vi "4155C Thermopower Heater ON Config SMUs.vi"(0 "VISA resource name in":refnum<visa-resource-name>, 1 "sweep method":u16(ring) items=["Continuous", "Pulsed"], 2 "Gate mode":u16(ring) items=["Auto", "Limited", "Fixed"], 3 "Gate Range":u8(slide)=6 max=11 scale=0.0..11.0, 5 "Pulse period":dbl=0.005 min=0.005 max=1.0 step=0.0001 format="%.4f", 7 "Pulse width":dbl=0.0005 min=0.0005 max=0.1 step=0.0001 format="%.4f", 8 "Drain Standby":bool, 9 "Base voltage":dbl format="%^.4e", 10 "Gate Standby":bool, 11 "error in (no error)":errorcluster, 12 "SMU4":cluster{"on/off":bool, "Voltage":dbl} {"Voltage" min=-100.0 max=100.0 format="%.2f"}, 13 "Source/drain mode":u16(ring) items=["Auto", "Limited", "Fixed"], 14 "Source/drain Range":u8(slide)=6 max=11 scale=0.0..11.0) -> (4 "VISA Resource Name out":refnum<visa-resource-name>, 15 "error out":errorcluster)   [LabVIEW 2016]
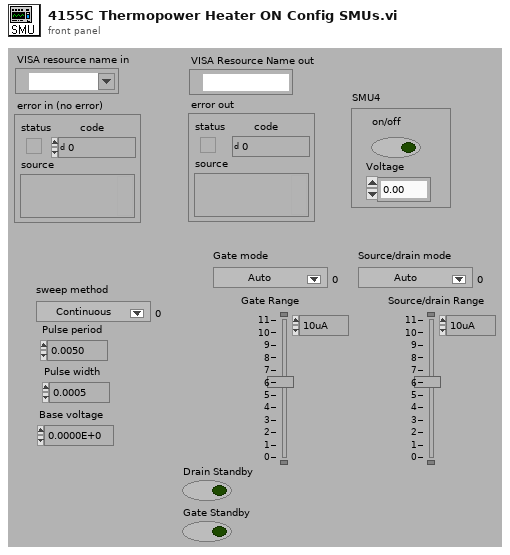
[diagram p1: front panel]
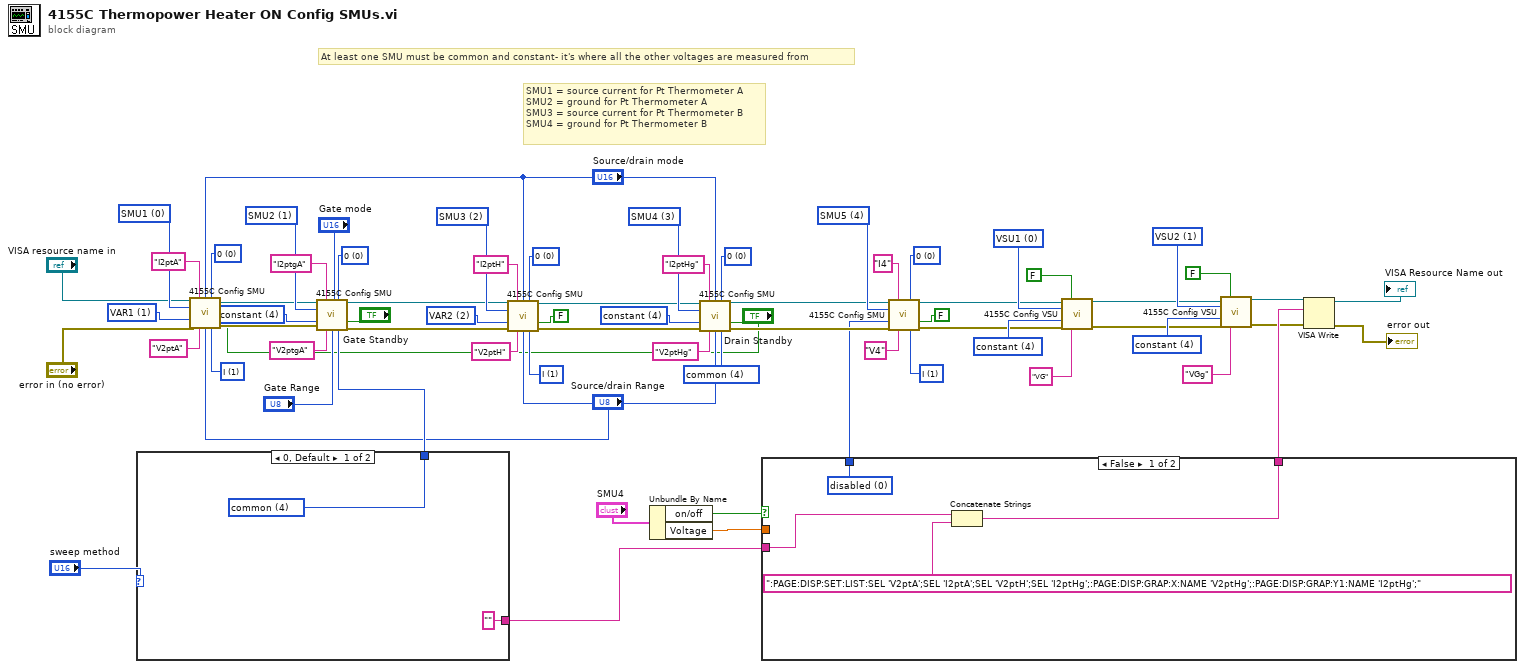
[diagram p0: block diagram]
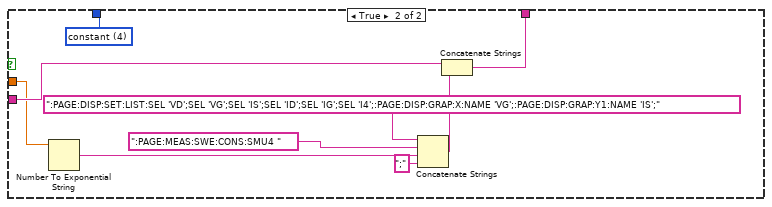
[diagram p2: hidden frame]
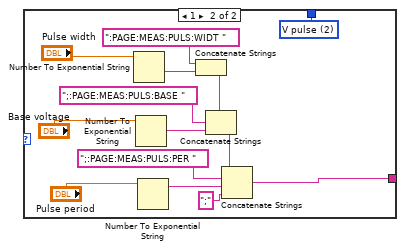
[diagram p3: hidden frame]
diagram:
  w7 = u32 4 items=["disabled  ", "VAR1  ", "VAR2  ", "VAR1'  ", "constant  "] ("function")
  w8 = u32 1 items=["VSU1  ", "VSU2  "] ("unit to configure")
  w13 = u32 4 items=["disabled  ", "VAR1  ", "VAR2  ", "VAR1'  ", "constant  "] ("function")
  w14 = u32 0 items=["VSU1  ", "VSU2  "] ("unit to configure")
  w29 = u32 0 items=["SMU1  ", "SMU2  ", "SMU3  ", "SMU4  ", "SMU5  ", "SMU6  "] ("unit to configure")
  w30 = u32 1 items=["disabled  ", "VAR1  ", "VAR2  ", "VAR1'  ", "constant  "] ("function")
  w32 = u32 0 items=["0  ", "10K Ohms  ", "100K Ohms  ", "1M Ohms  "] ("series resistance *")
  w33 = u32 1 items=["V  ", "I  ", "V pulse  ", "I pulse  ", "  common  "] ("mode")
  w49 = u32 1 items=["V  ", "I  ", "V pulse  ", "I pulse  ", "  common  "] ("mode")
  w50 = u32 0 items=["0  ", "10K Ohms  ", "100K Ohms  ", "1M Ohms  "] ("series resistance *")
  w52 = u32 4 items=["SMU1  ", "SMU2  ", "SMU3  ", "SMU4  ", "SMU5  ", "SMU6  "] ("unit to configure")
  w55 = u32 0 items=["0  ", "10K Ohms  ", "100K Ohms  ", "1M Ohms  "] ("series resistance *")
  w24 = u32 4 items=["disabled  ", "VAR1  ", "VAR2  ", "VAR1'  ", "constant  "] ("function")
  w57 = u32 1 items=["SMU1  ", "SMU2  ", "SMU3  ", "SMU4  ", "SMU5  ", "SMU6  "] ("unit to configure")
  w59 = u32 4 items=["V  ", "I  ", "V pulse  ", "I pulse  ", "  common  "] ("mode")
  w60 = u32 0 items=["0  ", "10K Ohms  ", "100K Ohms  ", "1M Ohms  "] ("series resistance *")
  w62 = u32 4 items=["disabled  ", "VAR1  ", "VAR2  ", "VAR1'  ", "constant  "] ("function")
  w63 = u32 3 items=["SMU1  ", "SMU2  ", "SMU3  ", "SMU4  ", "SMU5  ", "SMU6  "] ("unit to configure")
  w66 = u32 1 items=["V  ", "I  ", "V pulse  ", "I pulse  ", "  common  "] ("mode")
  w67 = u32 0 items=["0  ", "10K Ohms  ", "100K Ohms  ", "1M Ohms  "] ("series resistance *")
  w69 = u32 2 items=["disabled  ", "VAR1  ", "VAR2  ", "VAR1'  ", "constant  "] ("function")
  w70 = u32 2 items=["SMU1  ", "SMU2  ", "SMU3  ", "SMU4  ", "SMU5  ", "SMU6  "] ("unit to configure")
  # "SMU1 = source current for Pt Thermometer A\nSMU2 = ground for Pt Thermometer A\nSMU3 = source current for Pt Thermometer B\nSMU4 = ground for Pt Thermometer B"
  # "At least one SMU must be common and constant- it's where all the other voltages are measured from"
  n1 = case shown="0, Default" "sweep method" {
    tunnel: [w72 w86] -> w41
    tunnel: ["" w74] -> w21
    frame 0, Default {
      w72 = u32 4 items=["V  ", "I  ", "V pulse  ", "I pulse  ", "  common  "] ("mode")
    }
    frame 1 {
      w86 = u32 2 items=["V  ", "I  ", "V pulse  ", "I pulse  ", "  common  "] ("mode")
      n2 = Number To Exponential String(number="Pulse width") -> (E-format string=w82:string)  [unwired: 3 out]
      n3 = Number To Exponential String(number="Base voltage") -> (E-format string=w78:string)  [unwired: 3 out]
      n4 = Number To Exponential String(number="Pulse period") -> (E-format string=w75:string)  [unwired: 3 out]
      n5 = Concatenate Strings(":PAGE:MEAS:PULS:WIDT " ("Substring"), w82) -> (w80:string)
      n6 = Concatenate Strings(w80, ";:PAGE:MEAS:PULS:BASE " ("Substring"), w78) -> (w76:string)
      n7 = Concatenate Strings(w76, ";:PAGE:MEAS:PULS:PER " ("Substring"), w75, ";" ("Substring")) -> (w74:string)
    }
  }
  n8 = call "4155C Config SMU.vi"("VISA session"="VISA resource name in", "I name (max 6 chars)"="I2ptA", "Range mode"="Source/drain mode", "series resistance *"=w32, "unit to configure"=w29, "function"=w30, "standby"="Drain Standby", "error in (no error)"="error in (no error)", "V name (max 6 chars)"="V2ptA", "Range"="Source/drain Range", "mode"=w33) -> ("dup VISA resource name"=w27:refnum<visa-resource-name>, "error out"=w28:errorcluster)  [unwired: 3 out]
  n9 = call "4155C Config SMU.vi"("VISA session"=w27, "I name (max 6 chars)"="I2ptgA", "Range mode"="Gate mode", "series resistance *"=w55, "unit to configure"=w57, "function"=w24, "standby"="Gate Standby", "error in (no error)"=w28, "V name (max 6 chars)"="V2ptgA", "Range"="Gate Range", "mode"=w41) -> ("dup VISA resource name"=w38:refnum<visa-resource-name>, "error out"=w37:errorcluster)  [unwired: 3 out]
  n10 = call "4155C Config SMU.vi"("VISA session"=w38, "I name (max 6 chars)"="I2ptH", "Range mode"="Source/drain mode", "series resistance *"=w67, "unit to configure"=w70, "function"=w69, "standby"=FALSE, "error in (no error)"=w37, "V name (max 6 chars)"="V2ptH", "Range"="Source/drain Range", "mode"=w66) -> ("dup VISA resource name"=w46:refnum<visa-resource-name>, "error out"=w45:errorcluster)  [unwired: 3 out]
  n11 = Unbundle By Name("SMU4") -> ("on/off"=w19:bool, "Voltage"=w20:dbl)
  n12 = call "4155C Config SMU.vi"("VISA session"=w46, "I name (max 6 chars)"="I2ptHg", "Range mode"="Source/drain mode", "series resistance *"=w60, "unit to configure"=w63, "function"=w62, "standby"="Drain Standby", "error in (no error)"=w45, "V name (max 6 chars)"="V2ptHg", "Range"="Source/drain Range", "mode"=w59) -> ("dup VISA resource name"=w35:refnum<visa-resource-name>, "error out"=w36:errorcluster)  [unwired: 3 out]
  n13 = case shown="False" w19 {
    tunnel: w21 -> [w89 w99]
    tunnel: [w88 w98] -> w17
    tunnel: w20 -> [_ w96]
    tunnel: [w87 w97] -> w16
    frame False {
      w87 = u32 0 items=["disabled  ", "VAR1  ", "VAR2  ", "VAR1'  ", "constant  "] ("function")
      n14 = Concatenate Strings(w89, ":PAGE:DISP:SET:LIST:SEL 'V2ptA';SEL 'I2ptA';SEL 'V2ptH';SEL 'I2ptHg';:PAGE:DISP:GRAP:X:NAME 'V2ptHg';:PAGE:DISP:GRAP:Y1:NAME 'I2ptHg';" ("write buffer (\"\")")) -> (w88:string)
    }
    frame True {
      w97 = u32 4 items=["disabled  ", "VAR1  ", "VAR2  ", "VAR1'  ", "constant  "] ("function")
      n15 = Number To Exponential String(number=w96) -> (E-format string=w94:string)  [unwired: 3 out]
      n16 = Concatenate Strings(":PAGE:DISP:SET:LIST:SEL 'VD';SEL 'VG';SEL 'IS';SEL 'ID';SEL 'IG';SEL 'I4';:PAGE:DISP:GRAP:X:NAME 'VG';:PAGE:DISP:GRAP:Y1:NAME 'IS';" ("write buffer (\"\")"), ":PAGE:MEAS:SWE:CONS:SMU4 " ("write buffer (\"\")"), w94, ";" ("Substring")) -> (w92:string)
      n17 = Concatenate Strings(w99, w92) -> (w98:string)
    }
  }
  n18 = call "4155C Config SMU.vi"("VISA session"=w35, "I name (max 6 chars)"="I4", "series resistance *"=w50, "unit to configure"=w52, "function"=w16, "standby"=FALSE, "error in (no error)"=w36, "V name (max 6 chars)"="V4", "mode"=w49) -> ("dup VISA resource name"=w10:refnum<visa-resource-name>, "error out"=w9:errorcluster)  [unwired: 2 in, 3 out]
  n19 = call "4155C Config VSU.vi"("VISA session"=w10, "standby"=FALSE, "unit to configure"=w14, "function"=w13, "error in (no error)"=w9, "V name (max 6 chars)"="VG") -> ("dup VISA resource name"=w4:refnum<visa-resource-name>, "error out"=w3:errorcluster)  [unwired: 8 out]
  n20 = call "4155C Config VSU.vi"("VISA session"=w4, "standby"=FALSE, "unit to configure"=w8, "function"=w7, "error in (no error)"=w3, "V name (max 6 chars)"="VGg") -> ("dup VISA resource name"=w2:refnum<visa-resource-name>, "error out"=w1:errorcluster)  [unwired: 8 out]
  n21 = VISA Write(VISA resource name=w2, write buffer=w17, error in (no error)=w1) -> (VISA resource name out=→"VISA Resource Name out":refnum<visa-resource-name>, error out=→"error out":errorcluster)  [unwired: 1 out]
